vi "SumAroundPeak.vi"(10 "ZoomWidth":i32, 11 "spectrum in":dbl[](array[numeric])) -> (1 "SumOfPeak":dbl, 2 "MaxValue":dbl, 3 "MaxIndex":i32, 4 "ZoomSpectrum":dbl[](array[numeric]))   [LabVIEW 2018]
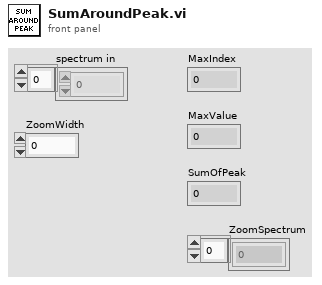
[diagram p1: front panel]
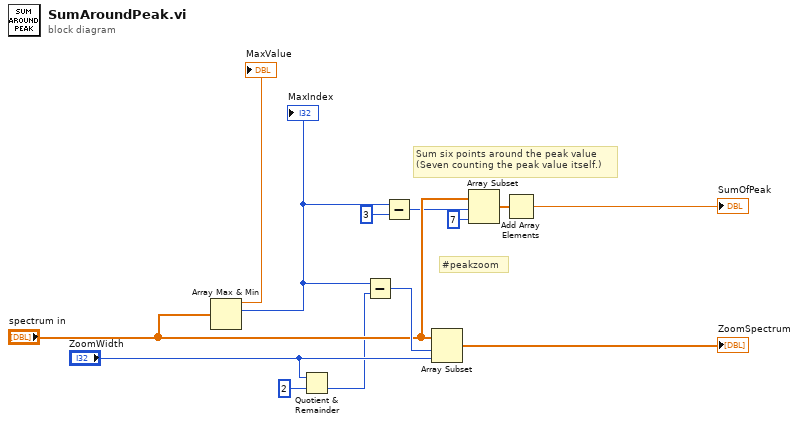
[diagram p0: block diagram]
diagram:
  # "#peakzoom"
  # "Sum six points around the peak value\n(Seven counting the peak value itself.)"
  n1 = Array Max & Min(array="spectrum in") -> (max value=→"MaxValue":dbl, max index (indices)=w5:i32)  [unwired: 2 out]
  "MaxIndex" <- w5
  n2 = Quotient & Remainder(x="ZoomWidth", y=2) -> (floor(x/y)=w3:i32)  [unwired: 1 out]
  n3 = Subtract(x=w5, y=w3) -> (x-y=w13:i32)
  n4 = Subtract(x=w5, y=3) -> (x-y=w7:i32)
  n5 = Array Subset(array="spectrum in", index=w13, length="ZoomWidth") -> (→"ZoomSpectrum":dbl[])
  n6 = Array Subset(array="spectrum in", index=w7, length=7) -> (w10:dbl[])
  n7 = Add Array Elements(numeric array=w10) -> (sum=→"SumOfPeak":dbl)
